vi "read_simple_data (SubVI).vi"(0 "number of samples per channel":i32=-1, 11 "data tasks":T1) -> (4 "output cluster":T1, 10 "sample rate":dbl, 14 "data":dbl[][](array[numeric]) format="%0.2f", 15 "Output data":i16[][](array[numeric]))   [LabVIEW 2018]
uses:
  <vilib>/DAQmx/read.llb/DAQmx Read (Analog 2D DBL NChan NSamp).vi
  <vilib>/DAQmx/miscellaneous.llb/DAQmx Fill In Error Info.vi
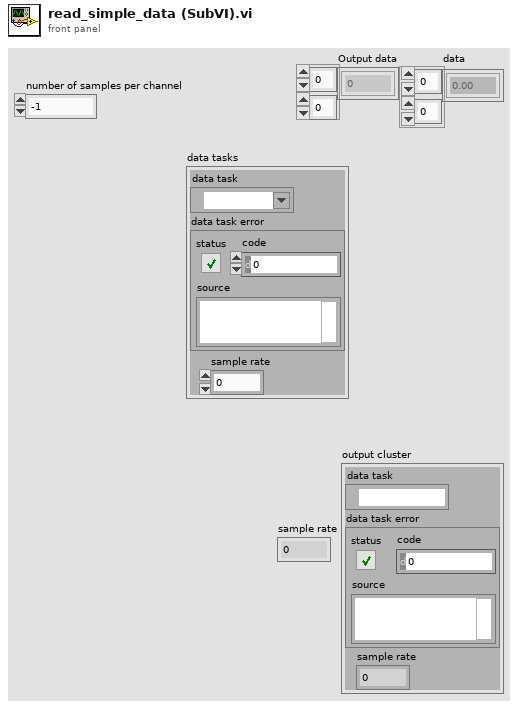
[diagram p1: front panel]
types:
  T1 = cluster{"data task":refnum<k21>, "data task error":errorcluster, "sample rate":dbl}
  T2 = cluster{"task out":refnum<k21>, "error out":errorcluster, "sample rate":dbl}
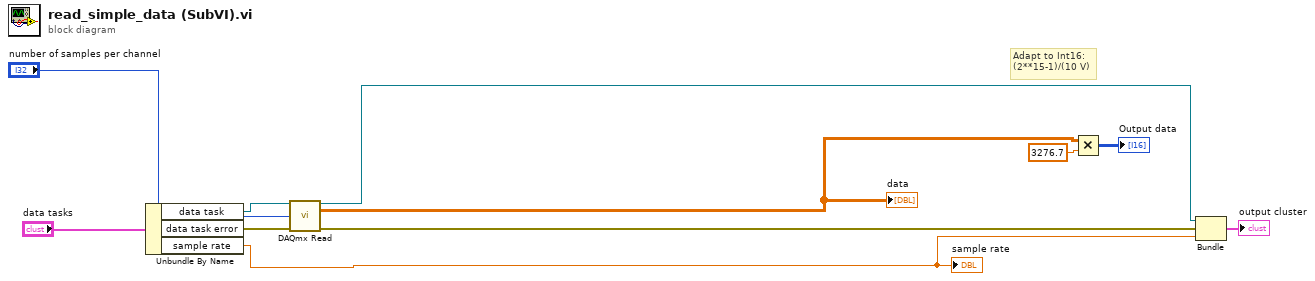
[diagram p0: block diagram]
diagram:
  # "Adapt to Int16: \n(2**15-1)/(10 V)"
  n1 = Unbundle By Name("data tasks") -> ("data task"=w6:refnum<k21>, "data task error"=w7:errorcluster, "sample rate"=w9:dbl)
  "sample rate" <- w9
  n2 = call-poly <vilib>:"DAQmx Read.vi"("task/channels in"=w6, "number of samples per channel"="number of samples per channel", "error in"=w7) -> ("task out"=w5:refnum<k21>, "data"=w3:dbl[][], "error out"=w4:errorcluster)  [unwired: 10 in]
  "data" <- w3
  n3 = Multiply(x=w3, y=3276.7) -> (x*y=→"Output data":i16[][])
  n4 = Bundle("task out"=w5, "error out"=w4, "sample rate"=w9) -> (→"output cluster":T2)  [unwired: 1 in]
